vi "ALTS-2015 Edit User Info v1.0.vi"(6 "Users":string[](array[string]), 7 "Add(T)/Edit(F)":bool, 8 "error in (no error)":errorcluster, 10 "User Group":T1, 11 "User Name":string="Administrator") -> (0 "error out":errorcluster={"status"=TRUE, "code"=-603, "source"="Open Registry Key.vi"})   [LabVIEW 2013]
uses:
  Controls/ALTS-2015 User Group Enum2.ctl
  Controls/ALTS-2015 Poll Control Edit Info.ctl
  Controls/ALTS-2015 User Info.ctl
panel:
  out "Saved?":bool
  out "Administrator?":bool
  in  "Select User":u16(ring) items=["Administrator", "Charu"]
  out "Time":string
  out "Title":string
  in  "Confirm Password":string="Administrator"
  in  "New Password":string="Administrator"
  in  "Old Password":string="Administrator"
  in  "Cancel":bool
  in  "OK":bool
  in  "User Group":u16(ring) items=["Administrator", "Super User", "Operator"]
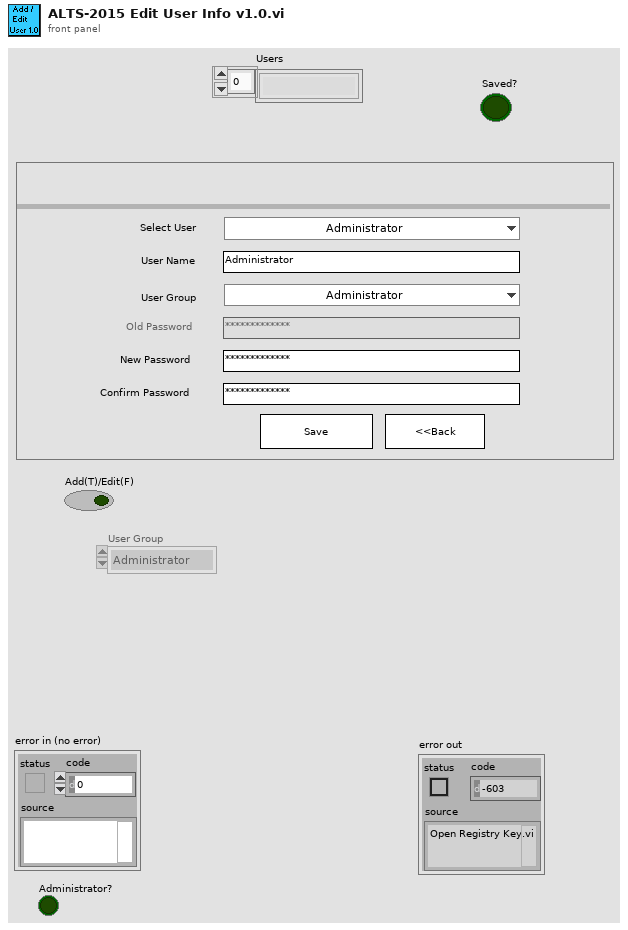
[diagram p1: front panel]
types:
  T1 = typedef "ALTS-2015 User Group Enum2.ctl" = enum16{"Administrator", "Super User", "Operator"}
  T2 = typedef "ALTS-2015 Poll Control Edit Info.ctl" = enum16{">Initialize", ">ReInitialize", ">Poll", ">NOP", ">On OK", ">On Cancel", ">Verify Password", ">About", ">Handle Error", ">Close Handles", ">UserChange", ">ReadUser", ">Exit"}
  T3 = typedef "ALTS-2015 User Info.ctl" = cluster{"User Name":string, "Password":string, "User Right":T1}
  T4 = enum16{"OK", "CANCEL", "ABORT", "RETRY", "IGNORE", "YES", "NO"}
  T5 = typedef "eventvkey.ctl" = enum16{"ASCII", "Enter", "Return", "Shift", "Ctrl", "Alt", "Cmd", "Opt", "Caps", "NumLock", "Clear", "Break", "Up", "Down", "Left", "Right", "Insert", "Delete", "Home", "End", "PageUp", "PageDown", "Escape", "Help", "Pause", "ScrollLock", "F1", "F2", "F3", "F4", "F5", "F6", "F7", "F8", "F9", "F10", "F11", "F12", "F13", "F14", "F15", "F16", "F17", "F18", "F19", "F20", "F21", "F22", "F23", "F24", "Play", "VolumeUp", "VolumeDown", "Mute", "Two Byte Char"}
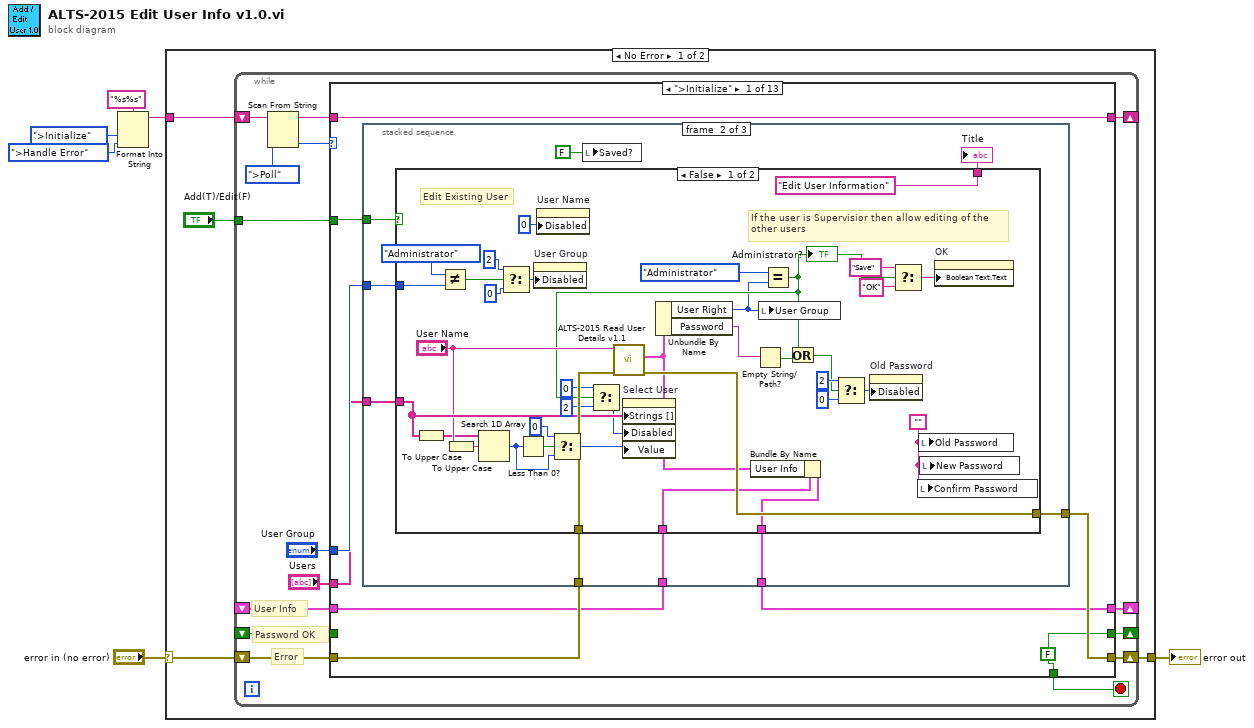
[diagram p0: block diagram]
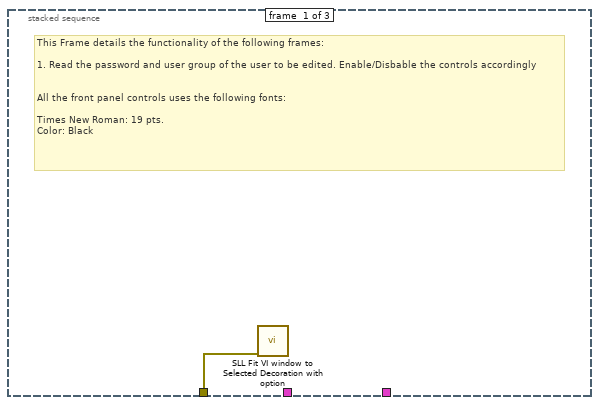
[diagram p2: hidden frame]
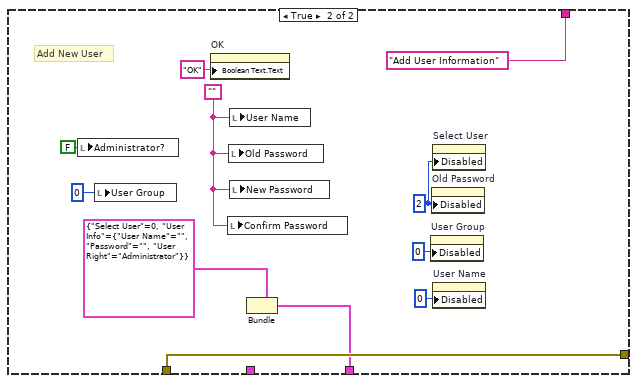
[diagram p3: hidden frame]
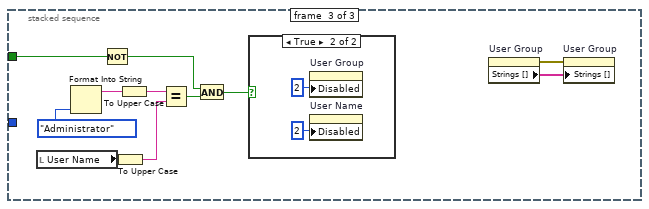
[diagram p4: hidden frame]
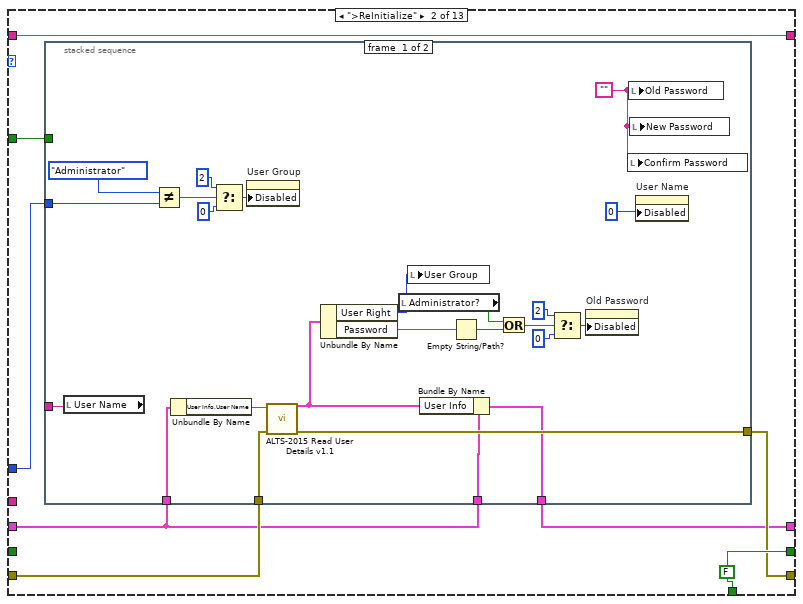
[diagram p6: hidden frame]
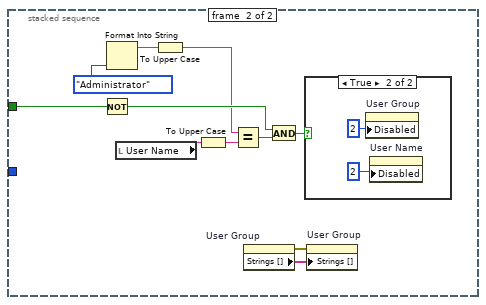
[diagram p7: hidden frame]
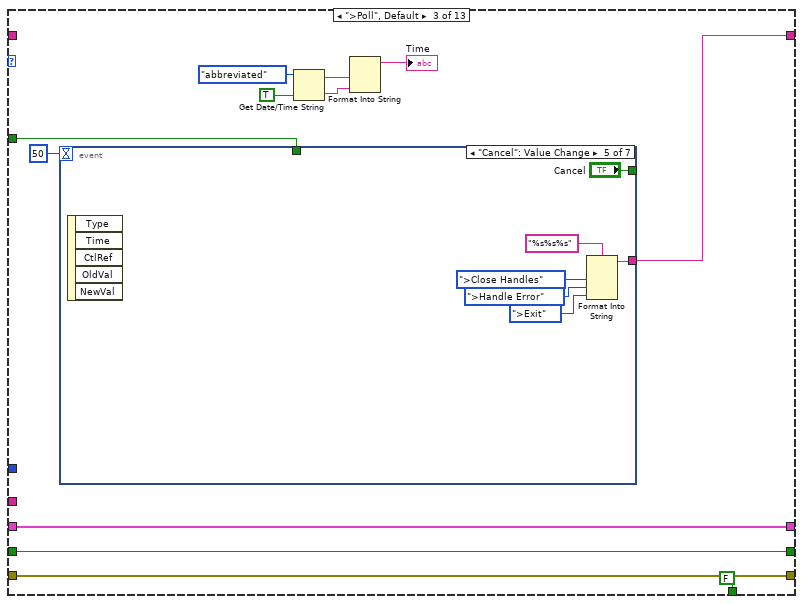
[diagram p9: hidden frame]
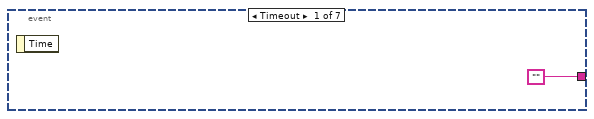
[diagram p10: hidden frame]
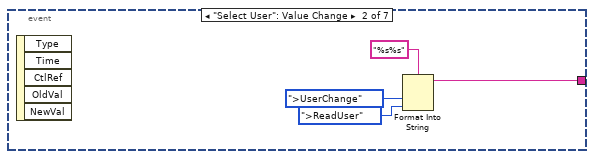
[diagram p11: hidden frame]
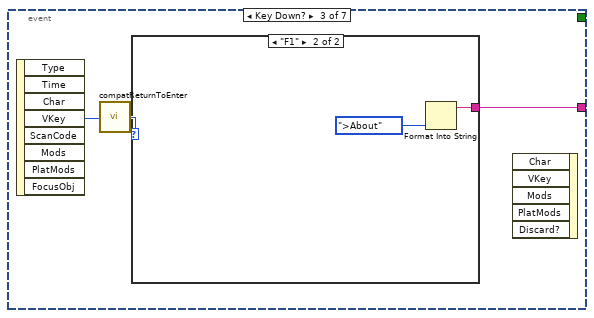
[diagram p12: hidden frame]
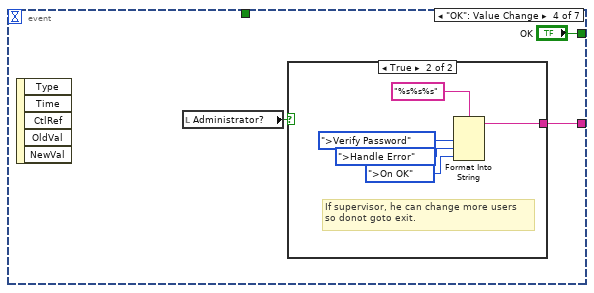
[diagram p14: hidden frame]
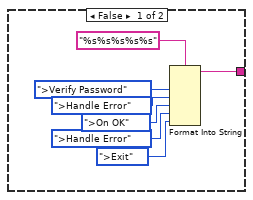
[diagram p15: hidden frame]
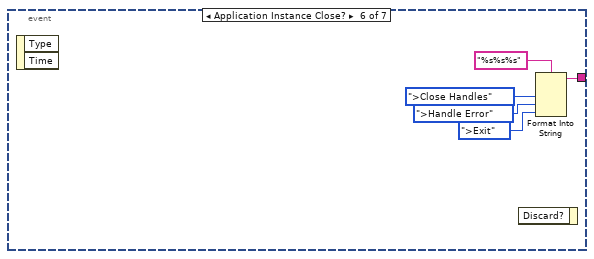
[diagram p16: hidden frame]
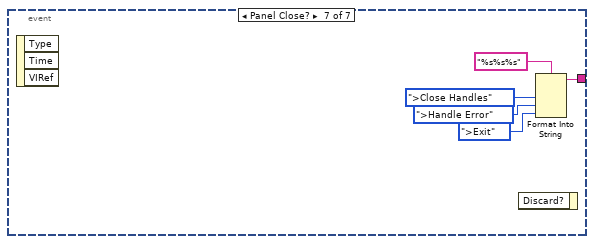
[diagram p17: hidden frame]
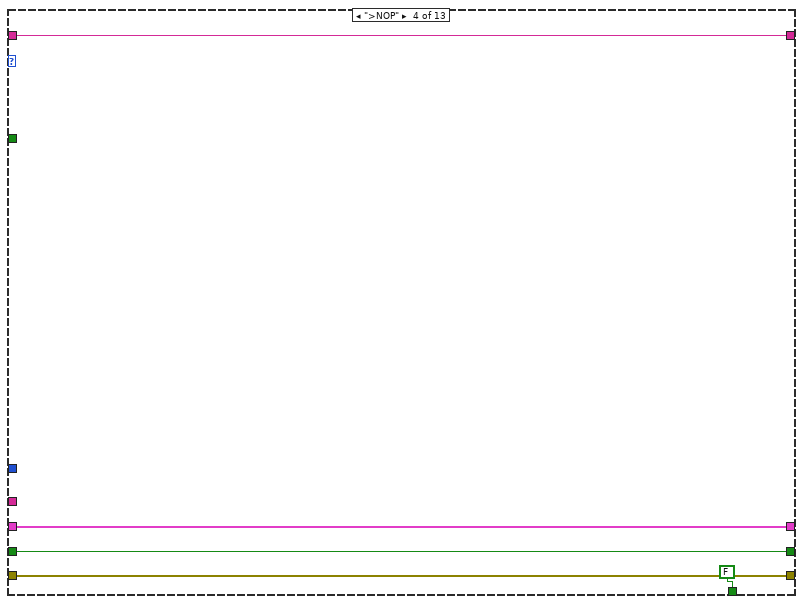
[diagram p18: hidden frame]
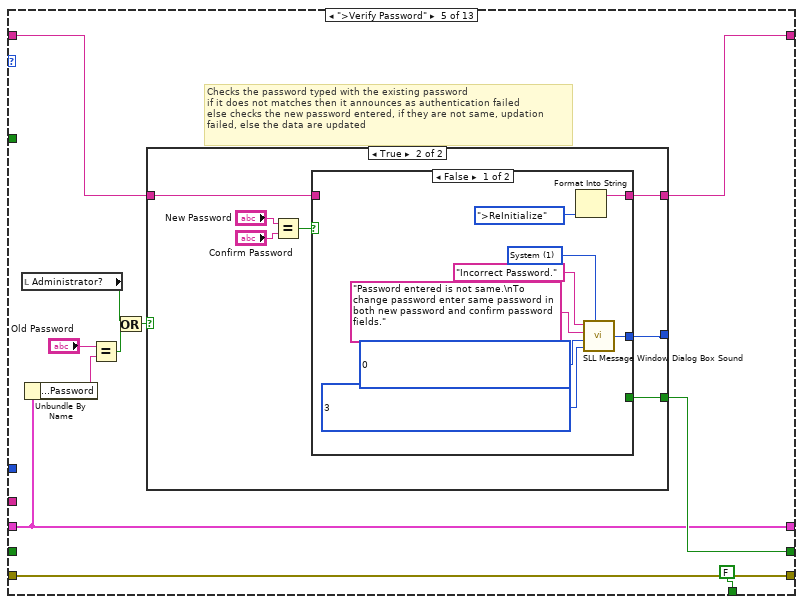
[diagram p19: hidden frame]
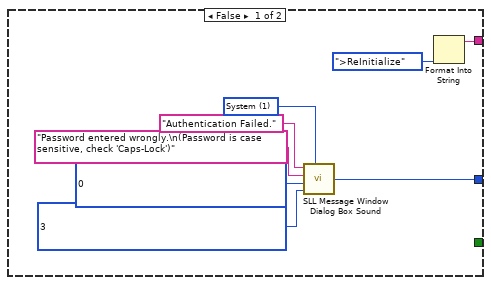
[diagram p20: hidden frame]
diagram:
  n1 = Format Into String(format string="%s%s", ALTS-2015_Poll_Control_Edit_Info.">Initialize" ("Enum"), ALTS-2015_Poll_Control_Edit_Info.">Handle Error" ("Enum")) -> (resulting string=w3:string)  [unwired: 2 in, 1 out]
  n2 = case shown="No Error" "error in (no error)" {
    selector: "error in (no error)" -> [w7 w428]
    tunnel: [w10 w428] -> w5
    tunnel: w3 -> [w8 _]
    frame No Error {
      n3 = while {
        shift-right: [w24] -> w10
        shift-left: w7 -> [w25]
        shift-right: [w21] -> _
        shift-left: _ -> [w22]
        shift-right: [w23] -> _
        shift-left: w8 -> [w18]
        tunnel: "Add(T)/Edit(F)" -> [w15]
        shift-right: [w12] -> _
        shift-left: _ -> [w11]
        stop <- w20 stop-if-true
        # "User Info"
        # "Password OK"
        # "Error"
        n4 = Scan From String(input string=w18, default 1=ALTS-2015_Poll_Control_Edit_Info.">Poll" ("Enum")) -> (remaining string=w19:string, output 1=w17:T2)  [unwired: 3 in, 2 out]
        n5 = case shown="\">Initialize\"" w17 {
          tunnel: w25 -> [w31 w110 w162 w207 w219 w248 w332 w337 w357 w362 w367 w389 w411]
          tunnel: [w32 w111 w162 w207 w219 w249 w332 _ w357 w362 w367 w389 w411] -> w24
          tunnel: w19 -> [w34 w113 _ w208 w215 w253 w333 w336 w358 w363 w368 w390 w406]
          tunnel: [w34 w113 w151 w208 w214 w253 w333 w335 w358 w363 w368 w390 w404] -> w23
          tunnel: w22 -> [_ _ w161 w205 _ w250 w330 w338 w355 w360 w365 w387 w409]
          tunnel: [w29 w112 w161 w205 w216 w250 w330 w338 w355 w360 w365 w387 w409] -> w21
          tunnel: [w29 w112 FALSE FALSE FALSE FALSE FALSE FALSE FALSE FALSE TRUE FALSE FALSE] -> w20
          tunnel: w15 -> [w33 w108 w153 _ _ w251 _ _ _ _ _ _ _]
          tunnel: "User Group" -> [w30 w109 _ _ _ _ _ _ _ _ _ _ _]
          tunnel: "Users" -> [w28 _ _ _ _ w247 _ _ _ _ _ w379 _]
          tunnel: [w27 w107 w152 w204 w210 w245 w329 w334 w353 w359 w364 w376 w407] -> w12
          tunnel: w11 -> [w26 w106 w152 w204 w210 w246 w329 w334 w353 w359 w364 w377 w407]
          frame ">Initialize" {
            w29 = FALSE
            n6 = stacked-sequence {
              tunnel: w33 -> [_ w44 w97]
              tunnel: w31 -> [w35 w43 _]
              tunnel: [_ w42 _] -> w32
              tunnel: w30 -> [_ w41 _]
              tunnel: w28 -> [_ w39 _]
              tunnel: [_ w38 _] -> w27
              tunnel: w26 -> [_ w37 _]
              frame #0 {
                # "This Frame details the functionality of the following frames:\n\n1. Read the password and user group of the user to be edited. Enable/Disbable the controls accordingly\n\n\nAll the front panel controls uses the following fonts:\n\nTimes New Roman: 19 pts.\nColor: Black"
                n7 = call <userlib>:"SLL Fit VI window to Selected Decoration with option.vi"("error in (no error)"=w35) -> ()  [unwired: 9 in, 2 out]
              }
              frame #1 {
                n8 = case shown="False" w44 {
                  tunnel: w43 -> [w77 w91]
                  tunnel: [w76 w91] -> w42
                  tunnel: w41 -> [w75 _]
                  tunnel: ["Edit User Information" ("Title") "Add User Information" ("Title")] -> w40
                  tunnel: w39 -> [w63 _]
                  tunnel: [w49 w84] -> w38
                  tunnel: w37 -> [w48 _]
                  frame False {
                    w81 = ""
                    # "If the user is Supervisior then allow editing of the\nother users"
                    # "Edit Existing User"
                    n9 = To Upper Case(1:w63) -> (0:w50:string[])
                    n10 = Not Equal?(x=ALTS-2015_User_Group_Enum2."Administrator" ("User Group"), y=w75) -> (x != y?=w70:bool)
                    n11 = To Upper Case(1:"User Name") -> (0:w51:string)
                    n12 = Search 1D Array(1D array=w50, element=w51) -> (index of element=w60:i32)  [unwired: 1 in]
                    n13 = Select(t=u8 2 ("Disabled"), s=w70, f=u8 0 ("Disabled")) -> (s? t:f=w73:u8)
                    n14 = Less Than 0?(x=w60) -> (x < 0?=w61:bool)
                    n15 = property on="User Group" class="Ring (strict)"("Disabled"=w73) -> ()  [unwired: 2 in, 2 out]
                    n16 = property on="User Name" class="Str"("Disabled"=u8 0) -> ()  [unwired: 2 in, 2 out]
                    n17 = Select(t=0, s=w61, f=w60) -> (s? t:f=w58:i32)
                    n18 = call "ALTS-2015 Read User Details v1.1.vi"("error in (no error)"=w77, "User Name"="User Name") -> ("error out"=w76:errorcluster, "User Info"=w46:T3)  [unwired: 7 in, 1 out]
                    n19 = Unbundle By Name(w46) -> ("User Right"=w47:T1, "Password"=w67:string)
                    n20 = Bundle By Name(cluster=w48, "User Info"=w46) -> (w49:cluster{"Select User":u16, "User Info":T3})
                    n21 = Empty String/Path?(string/path=w67) -> (empty?=w57:bool)
                    n22 = local write "User Group"(w47) -> ()
                    n23 = Equal?(x=ALTS-2015_User_Group_Enum2."Administrator" ("User Right"), y=w47) -> (x = y?=w55:bool)
                    "Administrator?" <- w55
                    n24 = Select(t=u8 0 ("Disabled"), s=w55, f=u8 2 ("Disabled")) -> (s? t:f=w53:u8)
                    n25 = property on="Select User" class="Ring (strict)"("Strings []"=w63, "Disabled"=w53, "Value"=w58) -> ()  [unwired: 2 in, 2 out]
                    n26 = Or(x=w55, y=w57) -> (x .or. y?=w56:bool)
                    n27 = Select(t=u8 2 ("Disabled"), s=w56, f=u8 0 ("Disabled")) -> (s? t:f=w78:u8)
                    n28 = property on="Old Password" class="Str"("Disabled"=w78) -> ()  [unwired: 2 in, 2 out]
                    n29 = Select(t="Save" ("Title"), s=w55, f="OK" ("Title")) -> (s? t:f=w65:string)
                    n30 = local write "Confirm Password"(w81) -> ()
                    n31 = local write "Old Password"(w81) -> ()
                    n32 = local write "New Password"(w81) -> ()
                    n33 = property on="OK" class="Bool"("Boolean Text.Text"=w65) -> ()  [unwired: 2 in, 2 out]
                  }
                  frame True {
                    w87 = u8 2 ("Disabled")
                    w92 = ""
                    # "Add New User"
                    n34 = local write "Administrator?"(FALSE ("ADMIN?")) -> ()
                    n35 = local write "User Group"(u16 0) -> ()
                    n36 = property on="OK" class="Bool"("Boolean Text.Text"="OK") -> ()  [unwired: 2 in, 2 out]
                    n37 = local write "Confirm Password"(w92) -> ()
                    n38 = local write "Old Password"(w92) -> ()
                    n39 = local write "User Name"(w92) -> ()
                    n40 = local write "New Password"(w92) -> ()
                    n41 = Bundle(cluster=cluster{"Select User":u16, "User Info":T3} {"Select User"=0, "User Info"={"User Name"="", "Password"="", "User Right"=enum."Administrator"}}) -> (w84:cluster{"Select User":u16, "User Info":T3})  [unwired: 2 in]
                    n42 = property on="User Group" class="Ring (strict)"("Disabled"=u8 0) -> ()  [unwired: 2 in, 2 out]
                    n43 = property on="Old Password" class="Str"("Disabled"=w87) -> ()  [unwired: 2 in, 2 out]
                    n44 = property on="Select User" class="Ring (strict)"("Disabled"=w87) -> ()  [unwired: 2 in, 2 out]
                    n45 = property on="User Name" class="Str"("Disabled"=u8 0) -> ()  [unwired: 2 in, 2 out]
                  }
                }
                "Title" <- w40
                n46 = local write "Saved?"(FALSE ("Saved?")) -> ()
              }
              frame #2 {
                n47 = local read "User Name"() -> (w100:string)
                n48 = Format Into String(ALTS-2015_User_Group_Enum2."Administrator" ("User Right")) -> (resulting string=w94:string)  [unwired: 3 in, 1 out]
                n49 = Not(x=w97) -> (.not. x?=w96:bool)
                n50 = To Upper Case(1:w100) -> (0:w101:string)
                n51 = To Upper Case(1:w94) -> (0:w93:string)
                n52 = Equal?(x=w93, y=w101) -> (x = y?=w98:bool)
                n53 = And(x=w96, y=w98) -> (x .and. y?=w99:bool)
                n54 = case shown="True" w99 {
                  frame False {
                  }
                  frame True {
                    n55 = property on="User Group" class="Ring (strict)"("Disabled"=u8 2) -> ()  [unwired: 2 in, 2 out]
                    n56 = property on="User Name" class="Str"("Disabled"=u8 2) -> ()  [unwired: 2 in, 2 out]
                  }
                }
                n57 = property on="User Group" class="Enum (strict)"() -> (error out=w102:errorcluster, "Strings []"=w103:string[])  [unwired: 2 in, 1 out]
                n58 = property on="User Group" class="Ring (strict)"(error in=w102, "Strings []"=w103) -> ()  [unwired: 1 in, 2 out]
              }
            }
          }
          frame ">ReInitialize" {
            w112 = FALSE
            n59 = stacked-sequence {
              tunnel: w110 -> [w137 _]
              tunnel: [w136 _] -> w111
              tunnel: w109 -> [w135 _]
              tunnel: w108 -> [_ w144]
              tunnel: [w123 _] -> _
              tunnel: w106 -> [w119 _]
              tunnel: [w118 _] -> w107
              tunnel: w106 -> [w115 _]
              frame #0 {
                w134 = ""
                n60 = local read "User Name"() -> (w123:string)
                n61 = Not Equal?(x=ALTS-2015_User_Group_Enum2."Administrator" ("User Group"), y=w135) -> (x != y?=w126:bool)
                n62 = Unbundle By Name(w115) -> ("User Info.User Name"=w114:string)
                n63 = Select(t=u8 2 ("Disabled"), s=w126, f=u8 0 ("Disabled")) -> (s? t:f=w129:u8)
                n64 = property on="User Group" class="Enum (strict)"("Disabled"=w129) -> ()  [unwired: 2 in, 2 out]
                n65 = call "ALTS-2015 Read User Details v1.1.vi"("error in (no error)"=w137, "User Name"=w114) -> ("error out"=w136:errorcluster, "User Info"=w116:T3)  [unwired: 7 in, 1 out]
                n66 = Unbundle By Name(w116) -> ("User Right"=w117:T1, "Password"=w124:string)
                n67 = local read "Administrator?"() -> (w122:bool)
                n68 = local write "User Group"(w117) -> ()
                n69 = Bundle By Name(cluster=w119, "User Info"=w116) -> (w118:cluster{"Select User":u16, "User Info":T3})
                n70 = Empty String/Path?(string/path=w124) -> (empty?=w121:bool)
                n71 = Or(x=w122, y=w121) -> (x .or. y?=w120:bool)
                n72 = Select(t=u8 2 ("Disabled"), s=w120, f=u8 0 ("Disabled")) -> (s? t:f=w131:u8)
                n73 = property on="Old Password" class="Str"("Disabled"=w131) -> ()  [unwired: 2 in, 2 out]
                n74 = local write "Confirm Password"(w134) -> ()
                n75 = local write "Old Password"(w134) -> ()
                n76 = local write "New Password"(w134) -> ()
                n77 = property on="User Name" class="Str"("Disabled"=u8 0) -> ()  [unwired: 2 in, 2 out]
              }
              frame #1 {
                n78 = Not(x=w144) -> (.not. x?=w145:bool)
                n79 = Format Into String(ALTS-2015_User_Group_Enum2."Administrator" ("User Right")) -> (resulting string=w139:string)  [unwired: 3 in, 1 out]
                n80 = local read "User Name"() -> (w143:string)
                n81 = To Upper Case(1:w139) -> (0:w138:string)
                n82 = To Upper Case(1:w143) -> (0:w148:string)
                n83 = Equal?(x=w138, y=w148) -> (x = y?=w146:bool)
                n84 = property on="User Group" class="Enum (strict)"() -> (error out=w142:errorcluster, "Strings []"=w141:string[])  [unwired: 2 in, 1 out]
                n85 = And(x=w145, y=w146) -> (x .and. y?=w147:bool)
                n86 = case shown="True" w147 {
                  frame False {
                  }
                  frame True {
                    n87 = property on="User Group" class="Ring (strict)"("Disabled"=u8 2) -> ()  [unwired: 2 in, 2 out]
                    n88 = property on="User Name" class="Str"("Disabled"=u8 2) -> ()  [unwired: 2 in, 2 out]
                  }
                }
                n89 = property on="User Group" class="Ring (strict)"(error in=w142, "Strings []"=w141) -> ()  [unwired: 1 in, 2 out]
              }
            }
          }
          frame ">Poll", Default {
            n90 = event shown="[4] \"Cancel\": Value Change" {
              selector: _ -> [_ _ _ _ _ _ _]
              dyn-events: _ -> [_ _ _ _ _ _ _]
              timeout: 50 -> [_ _ _ _ _ _ _]
              tunnel: [_ _ _ "OK" "Cancel" _ _] -> _
              tunnel: ["" w166 w169 w174 w190 w196 w201] -> w151
              tunnel: w153 -> [_ _ _ _ _ _ _]
              event Timeout {
                n91 = event-data() -> ()  [unwired: 1 in, 1 out]
              }
              event "Select User": Value Change {
                n92 = event-data() -> ()  [unwired: 1 in, 5 out]
                n93 = Format Into String(format string="%s%s", ALTS-2015_Poll_Control_Edit_Info.">UserChange" ("Enum"), ALTS-2015_Poll_Control_Edit_Info.">ReadUser" ("Enum")) -> (resulting string=w166:string)  [unwired: 2 in, 1 out]
              }
              event Key Down? {
                n94 = event-data() -> ("VKey"=w168:T5)  [unwired: 1 in, 7 out]
                n95 = call <vilib>:"compatReturnToEnter.vi"("VKey"=w168) -> ("VKey"=w170:T5)
                n96 = case shown="\"F1\"" w170 {
                  tunnel: [_ w171] -> w169
                  frame "ASCII", Default {
                  }
                  frame "F1" {
                    n97 = Format Into String(ALTS-2015_Poll_Control_Edit_Info.">About" ("Enum")) -> (resulting string=w171:string)  [unwired: 3 in, 1 out]
                  }
                }
                n98 = event-data() -> ()  [unwired: 6 in, 1 out]
              }
              event "OK": Value Change {
                n99 = event-data() -> ()  [unwired: 1 in, 5 out]
                n100 = local read "Administrator?"() -> (w173:bool)
                n101 = case shown="True" w173 {
                  tunnel: [w181 w183] -> w174
                  frame False {
                    n102 = Format Into String(format string="%s%s%s%s%s", ALTS-2015_Poll_Control_Edit_Info.">Verify Password" ("Enum"), ALTS-2015_Poll_Control_Edit_Info.">Handle Error" ("Enum"), ALTS-2015_Poll_Control_Edit_Info.">On OK" ("Enum"), ALTS-2015_Poll_Control_Edit_Info.">Handle Error" ("Enum"), ALTS-2015_Poll_Control_Edit_Info.">Exit" ("Enum")) -> (resulting string=w181:string)  [unwired: 2 in, 1 out]
                  }
                  frame True {
                    # "If supervisor, he can change more users\nso donot goto exit."
                    n103 = Format Into String(format string="%s%s%s", ALTS-2015_Poll_Control_Edit_Info.">Verify Password" ("Enum"), ALTS-2015_Poll_Control_Edit_Info.">Handle Error" ("Enum"), ALTS-2015_Poll_Control_Edit_Info.">On OK" ("Enum")) -> (resulting string=w183:string)  [unwired: 2 in, 1 out]
                  }
                }
              }
              event "Cancel": Value Change {
                n104 = event-data() -> ()  [unwired: 1 in, 5 out]
                n105 = Format Into String(format string="%s%s%s", ALTS-2015_Poll_Control_Edit_Info.">Close Handles" ("Enum"), ALTS-2015_Poll_Control_Edit_Info.">Handle Error" ("Enum"), ALTS-2015_Poll_Control_Edit_Info.">Exit" ("Enum")) -> (resulting string=w190:string)  [unwired: 2 in, 1 out]
              }
              event Application Instance Close? {
                n106 = event-data() -> ()  [unwired: 1 in, 2 out]
                n107 = event-data() -> ()  [unwired: 2 in, 1 out]
                n108 = Format Into String(format string="%s%s%s", ALTS-2015_Poll_Control_Edit_Info.">Close Handles" ("Enum"), ALTS-2015_Poll_Control_Edit_Info.">Handle Error" ("Enum"), ALTS-2015_Poll_Control_Edit_Info.">Exit" ("Enum")) -> (resulting string=w196:string)  [unwired: 2 in, 1 out]
              }
              event Panel Close? {
                n109 = event-data() -> ()  [unwired: 1 in, 3 out]
                n110 = event-data() -> ()  [unwired: 2 in, 1 out]
                n111 = Format Into String(format string="%s%s%s", ALTS-2015_Poll_Control_Edit_Info.">Close Handles" ("Enum"), ALTS-2015_Poll_Control_Edit_Info.">Handle Error" ("Enum"), ALTS-2015_Poll_Control_Edit_Info.">Exit" ("Enum")) -> (resulting string=w201:string)  [unwired: 2 in, 1 out]
              }
            }
            n112 = Get Date/Time String(date format (0)=enum16{"short", "long", "abbreviated"}."abbreviated", want seconds? (F)=TRUE) -> (date string=w157:string, time string=w156:string)  [unwired: 1 in]
            n113 = Format Into String(w157, w156) -> (resulting string=→"Time":string)  [unwired: 3 in, 1 out]
          }
          frame ">NOP" {
          }
          frame ">Verify Password" {
            # "Checks the password typed with the existing password\nif it does not matches then it announces as authentication failed\nelse checks the new password entered, if they are not same, updation\nfailed, else the data are updated"
            n114 = local read "Administrator?"() -> (w213:bool)
            n115 = Unbundle By Name(w210) -> ("User Info.Password"=w209:string)
            n116 = Equal?(x="Old Password", y=w209) -> (x = y?=w212:bool)
            n117 = Or(x=w213, y=w212) -> (x .or. y?=w211:bool)
            n118 = case shown="True" w211 {
              tunnel: [w222 w231] -> _
              tunnel: [_ w230] -> w216
              tunnel: w215 -> [_ w229]
              tunnel: [w220 w228] -> w214
              frame False {
                w226 = 1 items=["Application", "System", "Task"] ("modality (0)")
                n119 = call <userlib>:"SLL Message Window Dialog Box Sound.vi"("Modality (0)"=w226, "Icon (0:None)"=3 ("icon (0:None)"), "Buttons (0:OK)"=0 ("buttons (0:OK)"), "Message (\"\")"="Password entered wrongly.\n(Password is case sensitive, check 'Caps-Lock')" ("window title (\"\")"), "Window Title (\"\")"="Authentication Failed." ("window title (\"\")")) -> ("Button Pressed"=w222:T4)  [unwired: 1 in]
                n120 = Format Into String(ALTS-2015_Poll_Control_Edit_Info.">ReInitialize" ("Enum")) -> (resulting string=w220:string)  [unwired: 3 in, 1 out]
              }
              frame True {
                n121 = Equal?(x="New Password", y="Confirm Password") -> (x = y?=w232:bool)
                n122 = case shown="False" w232 {
                  tunnel: [w237 _] -> w231
                  tunnel: [_ TRUE] -> w230
                  tunnel: w229 -> [_ w243]
                  tunnel: [w235 w243] -> w228
                  frame False {
                    w241 = 1 items=["Application", "System", "Task"] ("modality (0)")
                    n123 = Format Into String(ALTS-2015_Poll_Control_Edit_Info.">ReInitialize" ("Enum")) -> (resulting string=w235:string)  [unwired: 3 in, 1 out]
                    n124 = call <userlib>:"SLL Message Window Dialog Box Sound.vi"("Modality (0)"=w241, "Icon (0:None)"=3 ("icon (0:None)"), "Buttons (0:OK)"=0 ("buttons (0:OK)"), "Message (\"\")"="Password entered is not same.\nTo change password enter same password in both new password and confirm password fields." ("window title (\"\")"), "Window Title (\"\")"="Incorrect Password." ("window title (\"\")")) -> ("Button Pressed"=w237:T4)  [unwired: 1 in]
                  }
                  frame True {
                  }
                }
              }
            }
          }
          frame ">On OK" {
            n125 = case shown="False" w251 {
              selector: w251 -> [w256 _]
              tunnel: w250 -> [w259 w281]
              tunnel: w248 -> [w258 w280]
              tunnel: [w257 w279] -> w249
              tunnel: w247 -> [_ w278]
              tunnel: w246 -> [w255 w277]
              tunnel: [w254 w277] -> w245
              frame False {
                # "Edit Exisiting User"
                n126 = case "Valid Password ?" shown="True" w259 {
                  tunnel: w258 -> [w261 w274]
                  tunnel: [w261 w275] -> w257
                  tunnel: w256 -> [_ w276]
                  tunnel: w255 -> [w260 w273]
                  tunnel: [w260 w272] -> w254
                  frame False {
                    w262 = ""
                    # "Password Not OK"
                    n127 = local write "Confirm Password"(w262) -> ()
                    n128 = local write "Old Password"(w262) -> ()
                    n129 = local write "New Password"(w262) -> ()
                  }
                  frame True {
                    # "Password OK"
                    n130 = local read "New Password"() -> (w265:string)
                    n131 = local read "User Name"() -> (w271:string)
                    n132 = local read "User Group"() -> (w264:u16)
                    n133 = Unbundle By Name(w273) -> ("User Info.User Name"=w266:string, "Select User"=w267:u16)
                    n134 = call "ALTS-2015 Delete User Information v1.0.vi"("error in (no error)"=w274, "Add(T)/Edit(F)"=w276, "User Name"=w266) -> ("error out"=w270:errorcluster)  [unwired: 7 in, 1 out]
                    n135 = call "ALTS-2015 Write Users v1.1.vi"("error in (no error)"=w270, "User Group"=w264, "Password"=w265, "User Name"=w271) -> ("error out"=w275:errorcluster)  [unwired: 7 in]
                    n136 = local read "Users"() -> (w269:string[])
                    n137 = Replace Array Subset(array=w269, new element=w271, index=w267) -> (w268:string[])
                    n138 = Bundle By Name(cluster=w273, "User Info.User Name"=w271, "User Info.Password"=w265, "User Info.User Right"=w264) -> (w272:cluster{"Select User":u16, "User Info":T3})
                    n139 = local write "Users"(w268) -> ()
                    n140 = property on="Select User" class="Ring (strict)"("Strings []"=w268) -> ()  [unwired: 2 in, 2 out]
                    "Saved?" <- TRUE ("Saved?")
                  }
                }
              }
              frame True {
                # "Add New User"
                n141 = case shown="True" w281 {
                  tunnel: w280 -> [w282 w295]
                  tunnel: [w282 w294] -> w279
                  tunnel: w278 -> [_ w287]
                  frame False {
                    w283 = ""
                    # "Password Not OK"
                    n142 = local write "Confirm Password"(w283) -> ()
                    n143 = local write "Old Password"(w283) -> ()
                    n144 = local write "New Password"(w283) -> ()
                  }
                  frame True {
                    # "Password OK"
                    n145 = local read "User Name"() -> (w292:string)
                    n146 = Format Into String(ALTS-2015_User_Group_Enum2."Administrator" ("User Right")) -> (resulting string=w285:string)  [unwired: 3 in, 1 out]
                    n147 = To Upper Case(1:w292) -> (0:w290:string)
                    n148 = To Upper Case(1:w287) -> (0:w288:string[])
                    n149 = To Upper Case(1:w285) -> (0:w284:string)
                    n150 = Empty String/Path?(string/path=w292) -> (empty?=w293:bool)
                    n151 = Search 1D Array(1D array=w288, element=w290) -> (index of element=w289:i32)  [unwired: 1 in]
                    n152 = Equal?(x=w290, y=w284) -> (x = y?=w291:bool)
                    n153 = case shown="True" w291 {
                      tunnel: w295 -> [w300 w323]
                      tunnel: [w299 w323] -> w294
                      tunnel: w293 -> [w298 _]
                      tunnel: w292 -> [w297 _]
                      tunnel: w289 -> [w296 _]
                      frame False {
                        n154 = case shown="True" w298 {
                          tunnel: w300 -> [w304 w322]
                          tunnel: [w303 w322] -> w299
                          tunnel: w297 -> [w302 _]
                          tunnel: [_ w316] -> _
                          tunnel: w296 -> [w301 _]
                          frame False {
                            # "User Name Not Null"
                            n155 = case shown="0, Default" w301 {
                              tunnel: w304 -> [w305 w315]
                              tunnel: [w305 w312] -> w303
                              tunnel: w302 -> [_ w311]
                              frame 0, Default {
                                w306 = 1 items=["Application", "System", "Task"] ("modality (0)")
                                n156 = call <userlib>:"SLL Message Window Dialog Box Sound.vi"("Modality (0)"=w306, "Icon (0:None)"=3 ("icon (0:None)"), "Buttons (0:OK)"=0 ("buttons (0:OK)"), "Message (\"\")"="User Name already exists" ("window title (\"\")"), "Window Title (\"\")"="Error..." ("window title (\"\")")) -> ()  [unwired: 1 in, 1 out]
                              }
                              frame -1 {
                                n157 = local read "New Password"() -> (w314:string)
                                n158 = local read "User Group"() -> (w313:u16)
                                n159 = call "ALTS-2015 Write Users v1.1.vi"("error in (no error)"=w315, "User Group"=w313, "Password"=w314, "User Name"=w311) -> ("error out"=w312:errorcluster)  [unwired: 7 in]
                              }
                            }
                          }
                          frame True {
                            w321 = 1 items=["Application", "System", "Task"] ("modality (0)")
                            # "User Name Is Null"
                            n160 = call <userlib>:"SLL Message Window Dialog Box Sound.vi"("Modality (0)"=w321, "Icon (0:None)"=3 ("icon (0:None)"), "Buttons (0:OK)"=0 ("buttons (0:OK)"), "Message (\"\")"="Invalid User Name.\nUser Name cannot be NULL." ("window title (\"\")"), "Window Title (\"\")"="Error..." ("window title (\"\")")) -> ("Button Pressed"=w316:T4)  [unwired: 1 in]
                          }
                        }
                      }
                      frame True {
                        w324 = 1 items=["Application", "System", "Task"] ("modality (0)")
                        n161 = call <userlib>:"SLL Message Window Dialog Box Sound.vi"("Modality (0)"=w324, "Icon (0:None)"=3 ("icon (0:None)"), "Buttons (0:OK)"=0 ("buttons (0:OK)"), "Message (\"\")"="ADMINISTRATOR User Name cannot be added" ("window title (\"\")"), "Window Title (\"\")"="Error..." ("window title (\"\")")) -> ()  [unwired: 1 in, 1 out]
                      }
                    }
                  }
                }
              }
            }
          }
          frame ">On Cancel" {
          }
          frame ">Handle Error" {
            n162 = case shown="Error" w337 {
              selector: w337 -> [_ w352]
              tunnel: [_ w343] -> _
              tunnel: w336 -> [w340 _]
              tunnel: [w340 w341] -> w335
              frame No Error {
              }
              frame Error {
                w346 = 1 items=["Application", "System", "Task"] ("modality (0)")
                n163 = Unbundle By Name(w352) -> ("source"=w351:string, "code"=w350:i32)
                n164 = Format Into String(format string="Error : %s\nError Code : %d", w351, w350) -> (resulting string=w348:string)  [unwired: 2 in, 1 out]
                n165 = call <userlib>:"SLL Message Window Dialog Box Sound.vi"("Modality (0)"=w346, "Icon (0:None)"=3 ("icon (0:None)"), "Buttons (0:OK)"=0 ("buttons (0:OK)"), "Message (\"\")"=w348, "Window Title (\"\")"="Error..." ("window title (\"\")")) -> ("Button Pressed"=w343:T4)  [unwired: 1 in]
                n166 = Format Into String(ALTS-2015_Poll_Control_Edit_Info.">Exit" ("Enum")) -> (resulting string=w341:string)  [unwired: 3 in, 1 out]
              }
            }
          }
          frame ">About" {
            n167 = One Button Dialog(message="Help will Be Provided") -> ()  [unwired: 1 in, 1 out]
          }
          frame ">Close Handles" {
          }
          frame ">Exit" {
          }
          frame ">ReadUser" {
            w372 = ""
            n168 = Format Into String(ALTS-2015_User_Group_Enum2."Administrator" ("User Right")) -> (resulting string=w370:string)  [unwired: 3 in, 1 out]
            n169 = To Upper Case(1:w370) -> (0:w369:string)
            n170 = Index Array(array=w379, index="Select User") -> (element=w384:string)
            n171 = To Upper Case(1:w384) -> (0:w385:string)
            n172 = call "ALTS-2015 Read User Details v1.1.vi"("User Name"=w384) -> ("User Info"=w386:T3, "User Name Out"=w378:string)  [unwired: 8 in, 1 out]
            n173 = Equal?(x=w369, y=w385) -> (x = y?=w383:bool)
            n174 = Unbundle By Name(w386) -> ("User Right"=w374:T1)  [unwired: 1 out]
            n175 = Select(t=2, s=w383, f=0) -> (s? t:f=w380:i32)
            n176 = local write "User Name"(w378) -> ()
            n177 = Bundle By Name(cluster=w377, "User Info"=w386, "Select User"="Select User") -> (w376:cluster{"Select User":u16, "User Info":T3})
            n178 = local write "User Group"(w374) -> ()
            n179 = property on="User Group" class="Ring (strict)"("Disabled"=w380) -> ()  [unwired: 2 in, 2 out]
            n180 = property on="User Name" class="Str"("Disabled"=w380) -> ()  [unwired: 2 in, 2 out]
            n181 = local write "Confirm Password"(w372) -> ()
            n182 = local write "Old Password"(w372) -> ()
            n183 = local write "New Password"(w372) -> ()
            n184 = local write "Saved?"(FALSE ("Saved?")) -> ()
          }
          frame ">UserChange" {
            # "If the selected user is administrator\ndonot allow to change the user name amd group"
            n185 = local read "Saved?"() -> (w403:bool)
            n186 = local read "New Password"() -> (w395:string)
            n187 = local read "User Name"() -> (w400:string)
            n188 = Unbundle By Name(w407) -> ("User Info.User Name"=w397:string)
            n189 = Unbundle By Name(w407) -> ("User Info.User Right"=w398:T1, "User Info.Password"=w396:string)
            n190 = Empty String/Path?(string/path=w395) -> (empty?=w392:bool)
            n191 = Not Equal?(x=w396, y=w395) -> (x != y?=w394:bool)
            n192 = Not(x=w392) -> (.not. x?=w391:bool)
            n193 = Not Equal?(x=w400, y=w397) -> (x != y?=w399:bool)
            n194 = Not Equal?(x="User Group", y=w398) -> (x != y?=w402:bool)
            n195 = Select(t=w394, s=w403, f=w391) -> (s? t:f=w393:bool)
            n196 = Compound Arithmetic op=OR(w399, w402, w393) -> (w401:bool)
            n197 = case "Value Changed" shown="True" w401 {
              tunnel: ["" w414] -> w405
              frame False {
              }
              frame True {
                w413 = 1 items=["Application", "System", "Task"] ("modality (0)")
                n198 = Format Into String(format string="%s%s%s", ALTS-2015_Poll_Control_Edit_Info.">Verify Password" ("Enum"), ALTS-2015_Poll_Control_Edit_Info.">Handle Error" ("Enum"), ALTS-2015_Poll_Control_Edit_Info.">On OK" ("Enum")) -> (resulting string=w416:string)  [unwired: 2 in, 1 out]
                n199 = call <userlib>:"SLL Message Window Dialog Box Sound.vi"("Modality (0)"=w413, "Icon (0:None)"=2 ("icon (0:None)"), "Buttons (0:OK)"=4 ("buttons (0:OK)"), "Message (\"\")"="User Information has changed\nDo you want to save the changes?" ("message (\"\")"), "Window Title (\"\")"="Data Changed!!!" ("window title (\"\")")) -> ("Button Pressed"=w423:T4)  [unwired: 1 in]
                n200 = Equal?(x=w423, y=T4."YES" ("button pressed")) -> (x = y?=w421:bool)
                n201 = Select(t=w416, s=w421, f="") -> (s? t:f=w414:string)
              }
            }
            n202 = Concatenate Strings(w405, w406) -> (w404:string)
          }
        }
      }
    }
    frame Error {
    }
  }
  "error out" <- w5
